vi "New Parameter File.vi"(8 "error in":errorcluster) -> (0 "error out":errorcluster, 3 "new parameter file":refnum<k24>)   [LabVIEW 2020, in "Ballard_429_Parameter_ni.lvlib"]
uses:
  Ballard_429_Parameter_ni.lvlib
  C:/Users/Administrator/Desktop/GIT/Ballard-Arinc-429-XML-Generator/Source/Assemblies/Ballard_429_Parameter_ni/bin/Debug/Ballard_429_Parameter_ni.dll
  Assemblies/Ballard_429_Parameter_ni/bin/Debug/Ballard_429_Parameter_ni.dll
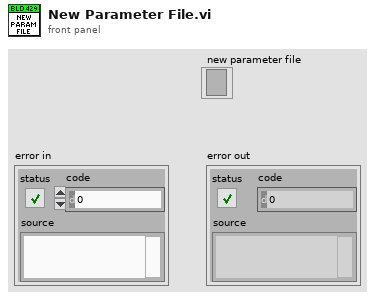
[diagram p1: front panel]
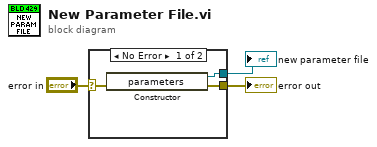
[diagram p0: block diagram]
diagram:
  n1 = case shown="No Error" "error in" {
    selector: "error in" -> [w4 _]
    tunnel: [w6 _] -> w3
    tunnel: [w5 _] -> w2
    frame No Error {
      n2 = constructor class="parameters"(error in=w4) -> (reference out=w6:refnum<k24>, error out=w5:errorcluster)  [unwired: 2 in, 1 out]
    }
    frame Error {
    }
  }
  "new parameter file" <- w3
  "error out" <- w2
